vi "Request Data.vi"(6 "Qualifier":string, 8 "error in":errorcluster, 9 "notifier":refnum<notifier>, 10 "Data to Send":string, 11 "CrossPoint in":refnum<class "CrossPoint.lvclass">) -> (0 "error out":errorcluster, 3 "CrossPoint out":refnum<class "CrossPoint.lvclass">)   [LabVIEW 2019, in "CrossPoint.lvlib" / "CrossPoint.lvclass"]
doc: "Data to Send is a required input that describes the measurement or query function to be performed\nQualifier is a secondary variable used in the event that specificity must be provided to the query function\n****Note****\nIf further specificity is required, the qualifier must be used in a comma delimited format to increase the overall variable count. Additional specificity must be provided by the child class and interpreted by the automated call.\n\nnotifier is a single variant notifier in which the instrument will send the data notification to the automated tool."
uses:
  Library/CrossPoint.lvclass
  builds/Instruments/Instruments.lvlibp/Library/Instruments.lvclass
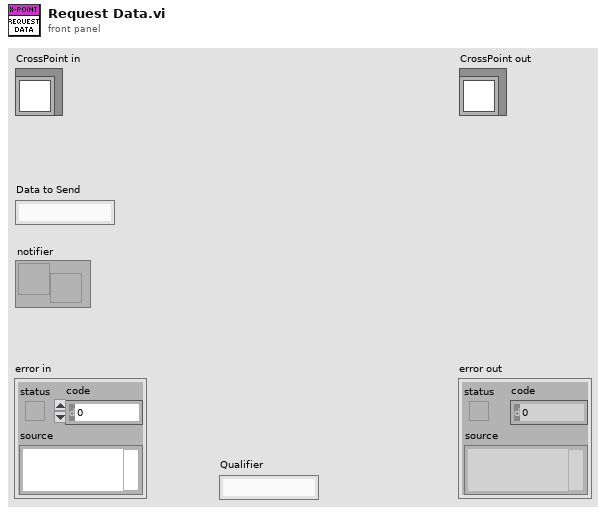
[diagram p1: front panel]
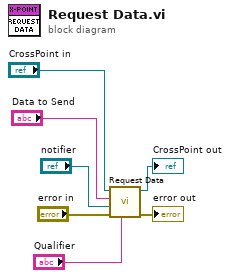
[diagram p0: block diagram]
diagram:
  n1 = call-parent "Request Data.vi"("Qualifier"="Qualifier", "error in"="error in", "notifier"="notifier", "Data to Send"="Data to Send", "Instruments in"="CrossPoint in") -> ("error out"=→"error out":errorcluster, "Instruments out"=→"CrossPoint out":refnum<class "CrossPoint.lvclass">)  [unwired: 5 in]
